vi "PJVS manual control GUI.vi"(11 "PJVS":T1={"PJVS type"=enum."AC-supraVOLTcontrol", "Status Refnum"=refnum, "AC-supraVOLTcontrol"={"IP address:port (0.0.0.0:0000)"="0.0.0.0:0000", "Timeouts"={"TCP Read & Write (ms)"=7000, "Sensors readout"=5000, "PJVS setup"=10000, "Nullmeter readout"=5000, "Multiplexer setup"=3000, "57XX setup"=15000, "Generator setup"=5000, "Synthesizer setup"=3000, "Sampler readout"=10000}, "Simulation mode"=FALSE, "Debug mode"=FALSE}, "NPL bias source"={"DataSocketCluster"={"Server Machine"="CZC105BD8M", "Client Machine"="localhost", "Data"="P2", "TimeStamp"=0.0, "Count"=1, "Target Process"="General Server"}}, "Manual PJVS"={"PJVS frequency (Hz)"=0.0, "Reference voltages (V)"=[], "File with PJVS voltages"=path ""}, "VTT PJVS"={"some VTT only property"=""}} {"NPL bias source"."DataSocketCluster"."TimeStamp" format="%.2f"}) -> ()   [LabVIEW 2020]
doc: "GUI to manally controll the PJVS. Relevant only for supracon PJVS or NPL Bias source."
uses:
  Type definitions/PJVS.ctl
  Type definitions/PJVS Type.ctl
  external libraries/acsvcontrol-driver/Public/Type Definitions/Timeouts.ctl
  external libraries/JV modified NPL Bias source/DataSocketCluster external.ctl
  <vilib>/Utility/error.llb/Error Cluster From Error Code.vi
  <vilib>/ErrorRing/Error Ring.xnode
  external libraries/varilib/varilib.lvlib
  external libraries/acsvcontrol-driver/ACSVcontrol-driver.lvlib
panel:
  in  "Tab Control":enum32{"Output parameters", "PJVS settings"}(tab)
  out "Status":string
  out "error out":errorcluster
  in  "Maximal signal amplitude (V)":dbl
  in  "Requested PJVS frequency (Hz)":dbl
  out "Set PJVS steps":u32
  in  "Requiested PJVS steps":u32
  out "PJVS reference voltages (1 period, V)":dbl[](array[numeric])
  out "Set frequency (Hz)":dbl
  out "Waveform Graph":dbl[](graph)
  in  "stop":bool
  in  "start":bool
  out "gui_elements":refnum<vi>[](array[refnum])
  in  "initialize":bool
  in  "quit":bool
  # "First ensure the PJVS is set correctly in tab \"PJVS settings\", next one can try set output\nin this tab."
  # "(If the amplitude is zero, DC 0 will be set on PJVS)"
  # "There is no sense trying to use \"Manual PJVS\" or \"VTT PJVS\" in this window."
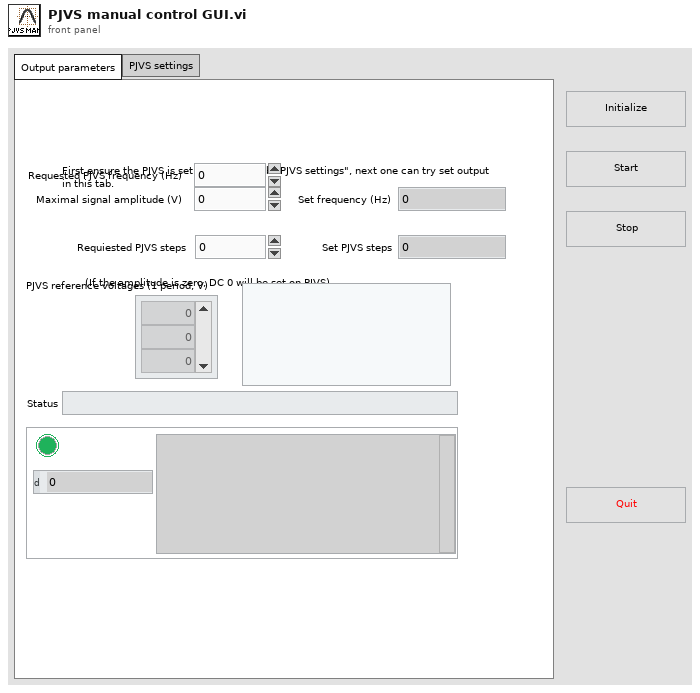
[diagram p1: front panel]
types:
  T1 = typedef "PJVS.ctl" = cluster{"PJVS type":T2, "Status Refnum":refnum<vi>, "AC-supraVOLTcontrol":cluster{"IP address:port (0.0.0.0:0000)":string, "Timeouts":T3, "Simulation mode":bool, "Debug mode":bool}, "NPL bias source":cluster{"DataSocketCluster":T4}, "Manual PJVS":cluster{"PJVS frequency (Hz)":dbl, "Reference voltages (V)":dbl[], "File with PJVS voltages":path}, "VTT PJVS":cluster{"some VTT only property":string}}
  T2 = typedef "PJVS Type.ctl" = enum16{"AC-supraVOLTcontrol", "JV modified NPL bias control", "Manual PJVS", "VTT PJVS"}
  T3 = typedef "ACSVcontrol-driver.lvlib/Timeouts.ctl" = cluster{"TCP Read & Write (ms)":i32, "Sensors readout":i32, "PJVS setup":i32, "Nullmeter readout":i32, "Multiplexer setup":i32, "57XX setup":i32, "Generator setup":i32, "Synthesizer setup":i32, "Sampler readout":i32}
  T4 = typedef "DataSocketCluster external.ctl" = cluster{"Server Machine":string, "Client Machine":string, "Data":string, "TimeStamp":dbl, "Count":i32, "Target Process":string}
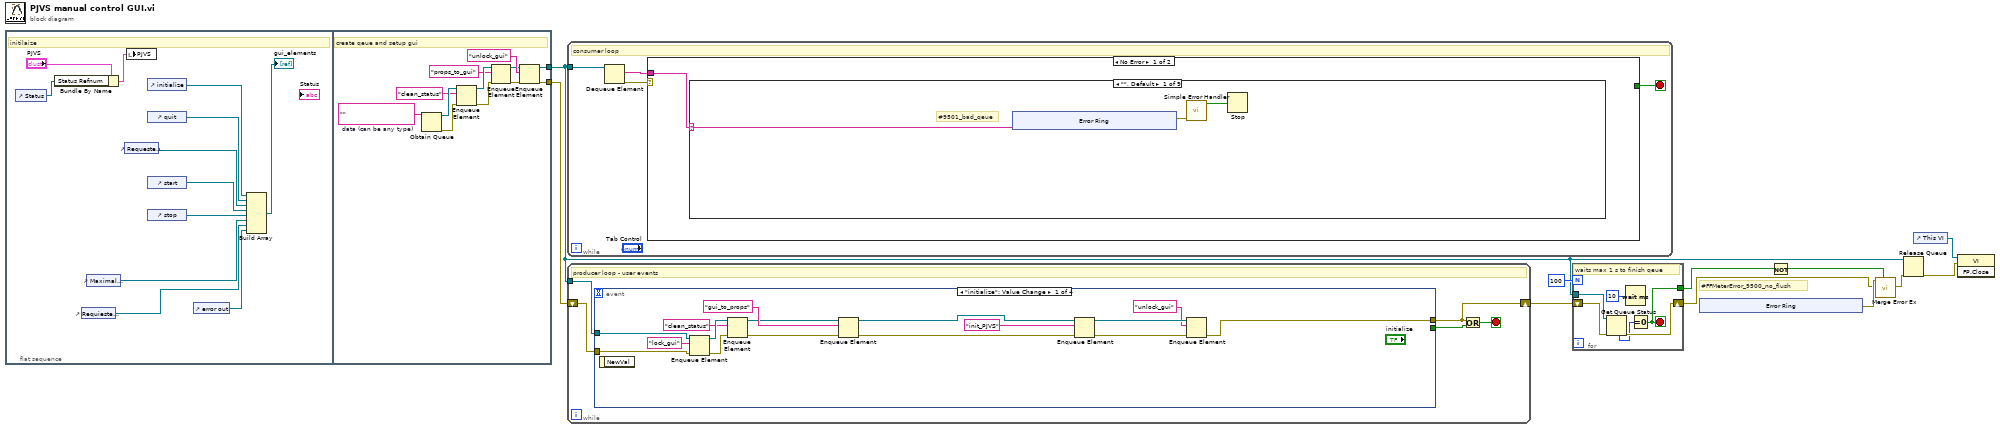
[diagram p0: block diagram]
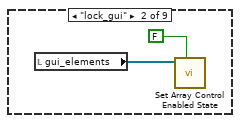
[diagram p2: hidden frame]
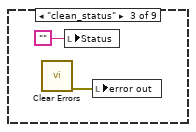
[diagram p3: hidden frame]
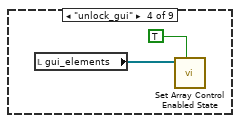
[diagram p4: hidden frame]
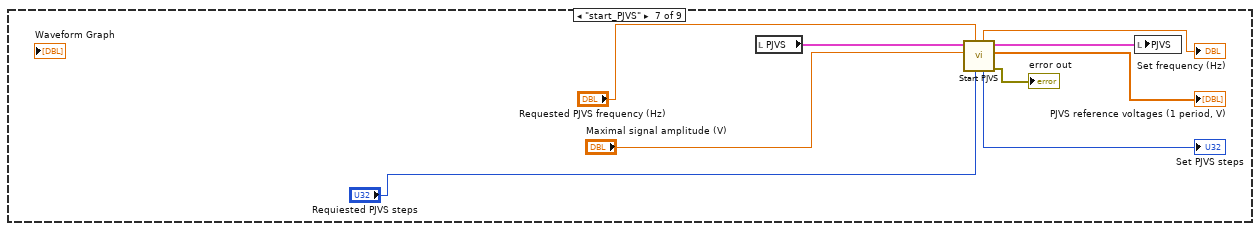
[diagram p7: hidden frame]
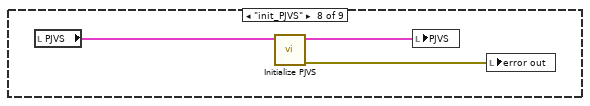
[diagram p8: hidden frame]
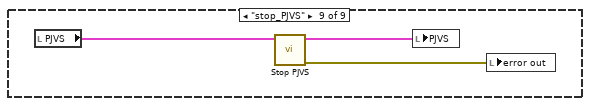
[diagram p9: hidden frame]
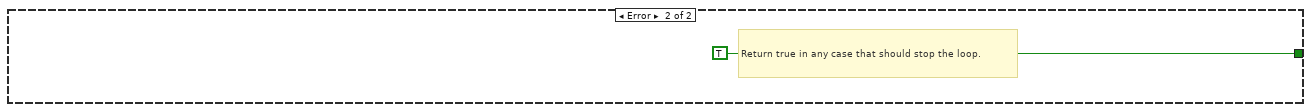
[diagram p10: hidden frame]
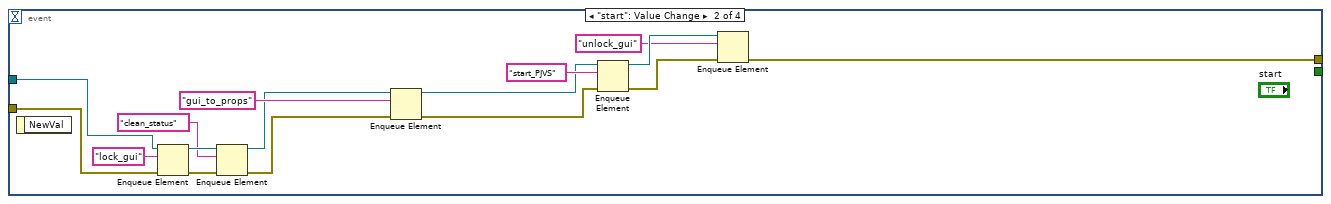
[diagram p11: hidden frame]
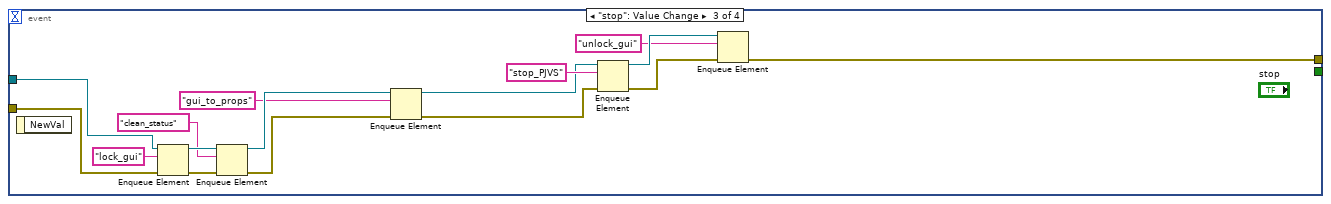
[diagram p12: hidden frame]
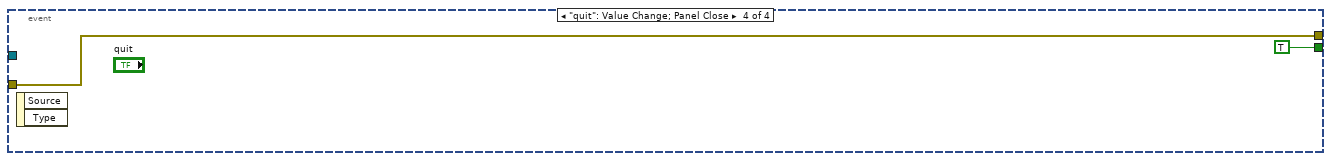
[diagram p13: hidden frame]
diagram:
  # "#FFMeterError_9500_no_flush"
  n1 = flat-sequence {
    tunnel: [w31] -> w4
    tunnel: [w29] -> w3
    frame #0 {
      # "initilaize"
      n2 = control-ref of="Status"() -> (w13:refnum<vi>)
      n3 = Bundle By Name(cluster="PJVS", "Status Refnum"=w13) -> (w14:T1)
      n4 = control-ref of="Requiested PJVS steps"() -> (w16:refnum<vi>)
      n5 = control-ref of="Maximal signal amplitude (V)"() -> (w17:refnum<vi>)
      n6 = control-ref of="Requested PJVS frequency (Hz)"() -> (w12:refnum<vi>)
      n7 = local write "PJVS"(w14) -> ()
      n8 = control-ref of="initialize"() -> (w23:refnum<vi>)
      n9 = control-ref of="quit"() -> (w22:refnum<vi>)
      n10 = control-ref of="start"() -> (w19:refnum<vi>)
      n11 = control-ref of="stop"() -> (w20:refnum<vi>)
      n12 = control-ref of="error out"() -> (w18:refnum<vi>)
      n13 = Build Array(w23, w22, w12, w19, w20, w17, w16, w18) -> (→"gui_elements":refnum<vi>[])
    }
    frame #1 {
      w30 = ""  # data (can be any type)
      # "create qeue and setup gui"
      n14 = Obtain Queue(element data type=w30) -> (queue out=w34:refnum<queue>, error out=w35:errorcluster)  [unwired: 4 in, 1 out]
      n15 = Enqueue Element(queue=w34, element="clean_status", error in (no error)=w35) -> (queue out=w27:refnum<queue>, error out=w28:errorcluster)  [unwired: 1 in, 1 out]
      n16 = Enqueue Element(queue=w27, element="props_to_gui", error in (no error)=w28) -> (queue out=w26:refnum<queue>, error out=w25:errorcluster)  [unwired: 1 in, 1 out]
      n17 = Enqueue Element(queue=w26, element="unlock_gui", error in (no error)=w25) -> (queue out=w31:refnum<queue>, error out=w29:errorcluster)  [unwired: 1 in, 1 out]
    }
  }
  n18 = while {
    tunnel: w4 -> [w39]
    stop <- w36 stop-if-true
    # "consumer loop"
    n19 = Dequeue Element(queue=w39) -> (element=w37:string, error out=w38:errorcluster)  [unwired: 2 in, 2 out]
    n20 = case shown="No Error" w38 {
      tunnel: w37 -> [w40 _]
      tunnel: [_ TRUE] -> w36
      frame No Error {
        n21 = case shown="\"\", Default" w40 {
          selector: w40 -> [w41 _ _ _ _ _ _ _ _]
          frame "", Default {
            # "#9501_bad_qeue"
            n22 = xnode "Error Ring"("parameter 0"=w41) -> ("error out"=w43:errorcluster)
            n23 = call <vilib>:"Simple Error Handler.vi"("error in (no error)"=w43) -> ("error?"=w42:bool)  [unwired: 4 in, 4 out]
            n24 = Stop(stop? (T)=w42) -> ()
          }
          frame "lock_gui" {
            n25 = local read "gui_elements"() -> (w52:refnum<vi>[])
            n26 = call "Set Array Control Enabled State.vi"("enabled (T)"=FALSE, "reference array in"=w52) -> ()  [unwired: 8 in, 2 out]
          }
          frame "clean_status" {
            n27 = call <vilib>:"Clear Errors.vi"() -> ("error out"=w53:errorcluster)  [unwired: 6 in, 1 out]
            n28 = local write "Status"("") -> ()
            n29 = local write "error out"(w53) -> ()
          }
          frame "unlock_gui" {
            n30 = local read "gui_elements"() -> (w56:refnum<vi>[])
            n31 = call "Set Array Control Enabled State.vi"("enabled (T)"=TRUE, "reference array in"=w56) -> ()  [unwired: 8 in, 2 out]
          }
          frame "props_to_gui" {
          }
          frame "gui_to_props" {
          }
          frame "start_PJVS" {
            n32 = local read "PJVS"() -> (w65:T1)
            n33 = call "Start PJVS.vi"("Requiested PJVS steps"="Requiested PJVS steps", "Requested PJVS frequency (Hz)"="Requested PJVS frequency (Hz)", "Maximal signal amplitude (V)"="Maximal signal amplitude (V)", "PJVS setup"=w65) -> ("error out"=→"error out":errorcluster, "PJVS reference voltages (1 period, V)"=→"PJVS reference voltages (1 period, V)":dbl[], "PJVS setup out"=w64:T1, "Set PJVS steps"=→"Set PJVS steps":u32, "Set frequency (Hz)"=→"Set frequency (Hz)":dbl)  [unwired: 3 in]
            n34 = local write "PJVS"(w64) -> ()
          }
          frame "init_PJVS" {
            n35 = local read "PJVS"() -> (w67:T1)
            n36 = call "Initialize PJVS.vi"("PJVS setup"=w67) -> ("error out"=w68:errorcluster, "PJVS setup out"=w66:T1)  [unwired: 9 in]
            n37 = local write "PJVS"(w66) -> ()
            n38 = local write "error out"(w68) -> ()
          }
          frame "stop_PJVS" {
            n39 = local read "PJVS"() -> (w69:T1)
            n40 = call "Stop PJVS.vi"("PJVS setup"=w69) -> ("error out"=w71:errorcluster, "PJVS setup out"=w70:T1)  [unwired: 9 in]
            n41 = local write "PJVS"(w70) -> ()
            n42 = local write "error out"(w71) -> ()
          }
        }
      }
      frame Error {
        # "Return true in any case that should stop the loop."
      }
    }
  }
  n43 = while {
    shift-right: [w73] -> w7
    shift-left: w3 -> [w76]
    tunnel: w4 -> [w77]
    stop <- w74 stop-if-true
    # "producer loop - user events"
    n44 = event shown="[0] \"initialize\": Value Change" {
      selector: _ -> [_ _ _ _]
      dyn-events: _ -> [_ _ _ _]
      timeout: _ -> [_ _ _ _]
      tunnel: w77 -> [w87 w103 w119 _]
      tunnel: w76 -> [w88 w104 w120 w127]
      tunnel: [w91 w107 w123 w127] -> w73
      tunnel: [_ _ _ TRUE ("cancel")] -> w75
      event "initialize": Value Change {
        n45 = event-data() -> ()  [unwired: 1 in, 1 out]
        n46 = Enqueue Element(queue=w87, element="lock_gui", error in (no error)=w88) -> (queue out=w84:refnum<queue>, error out=w85:errorcluster)  [unwired: 1 in, 1 out]
        n47 = Enqueue Element(queue=w84, element="clean_status", error in (no error)=w85) -> (queue out=w81:refnum<queue>, error out=w80:errorcluster)  [unwired: 1 in, 1 out]
        n48 = Enqueue Element(queue=w81, element="gui_to_props", error in (no error)=w80) -> (queue out=w78:refnum<queue>, error out=w79:errorcluster)  [unwired: 1 in, 1 out]
        n49 = Enqueue Element(queue=w78, element="init_PJVS", error in (no error)=w79) -> (queue out=w90:refnum<queue>, error out=w92:errorcluster)  [unwired: 1 in, 1 out]
        n50 = Enqueue Element(queue=w90, element="unlock_gui", error in (no error)=w92) -> (error out=w91:errorcluster)  [unwired: 1 in, 2 out]
      }
      event "start": Value Change {
        n51 = event-data() -> ()  [unwired: 1 in, 1 out]
        n52 = Enqueue Element(queue=w103, element="lock_gui", error in (no error)=w104) -> (queue out=w100:refnum<queue>, error out=w101:errorcluster)  [unwired: 1 in, 1 out]
        n53 = Enqueue Element(queue=w100, element="clean_status", error in (no error)=w101) -> (queue out=w97:refnum<queue>, error out=w96:errorcluster)  [unwired: 1 in, 1 out]
        n54 = Enqueue Element(queue=w97, element="gui_to_props", error in (no error)=w96) -> (queue out=w94:refnum<queue>, error out=w95:errorcluster)  [unwired: 1 in, 1 out]
        n55 = Enqueue Element(queue=w94, element="start_PJVS", error in (no error)=w95) -> (queue out=w106:refnum<queue>, error out=w108:errorcluster)  [unwired: 1 in, 1 out]
        n56 = Enqueue Element(queue=w106, element="unlock_gui", error in (no error)=w108) -> (error out=w107:errorcluster)  [unwired: 1 in, 2 out]
      }
      event "stop": Value Change {
        n57 = event-data() -> ()  [unwired: 1 in, 1 out]
        n58 = Enqueue Element(queue=w119, element="lock_gui", error in (no error)=w120) -> (queue out=w116:refnum<queue>, error out=w117:errorcluster)  [unwired: 1 in, 1 out]
        n59 = Enqueue Element(queue=w116, element="clean_status", error in (no error)=w117) -> (queue out=w113:refnum<queue>, error out=w114:errorcluster)  [unwired: 1 in, 1 out]
        n60 = Enqueue Element(queue=w113, element="gui_to_props", error in (no error)=w114) -> (queue out=w112:refnum<queue>, error out=w111:errorcluster)  [unwired: 1 in, 1 out]
        n61 = Enqueue Element(queue=w112, element="stop_PJVS", error in (no error)=w111) -> (queue out=w122:refnum<queue>, error out=w124:errorcluster)  [unwired: 1 in, 1 out]
        n62 = Enqueue Element(queue=w122, element="unlock_gui", error in (no error)=w124) -> (error out=w123:errorcluster)  [unwired: 1 in, 2 out]
      }
      event "quit": Value Change; Panel Close {
        n63 = event-data() -> ()  [unwired: 1 in, 2 out]
      }
    }
    n64 = Or(x=w73, y=w75) -> (x .or. y?=w74:bool)
  }
  n65 = for {
    N: 100 -> [_]
    tunnel: w4 -> [w133]
    shift-right: [w131] -> w8
    shift-left: w7 -> [w132]
    tunnel: [w128] -> w5
    stop <- w128 stop-if-true
    # "waits max 1 s to finish qeue"
    n66 = Get Queue Status(queue=w133, error in (no error)=w132) -> (error out=w131:errorcluster, # elements in queue=w129:i32)  [unwired: 1 in, 6 out]
    n67 = Wait (ms)(milliseconds to wait=u32 10) -> ()  [unwired: 1 out]
    n68 = Equal To 0?(x=w129) -> (x = 0?=w128:bool)
  }
  n69 = xnode "Error Ring"() -> ("error out"=w9:errorcluster)
  n70 = Not(x=w5) -> (.not. x?=w10:bool)
  n71 = call "Merge Error Ex.vi"("Is error? (False)"=w10, "main error in (no error)"=w8, "second error in"=w9) -> ("error out"=w6:errorcluster)  [unwired: 8 in]
  n72 = Release Queue(queue=w4, error in (no error)=w6) -> (error out=w1:errorcluster)  [unwired: 1 in, 2 out]
  n73 = control-ref of="This VI"() -> (w2:refnum<vi>)
  n74 = invoke class="VI" method="FP.Close"(reference=w2, error in=w1) -> ()  [unwired: 1 in, 3 out]
